vi "Untitled 2.vi"(7 "Before":dbl[][](array[numeric]), 11 "After":dbl[][](array[numeric])) -> (6 "Numeric":dbl)   [LabVIEW 2016]
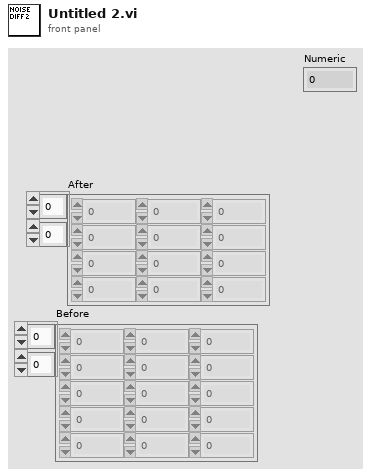
[diagram p1: front panel]
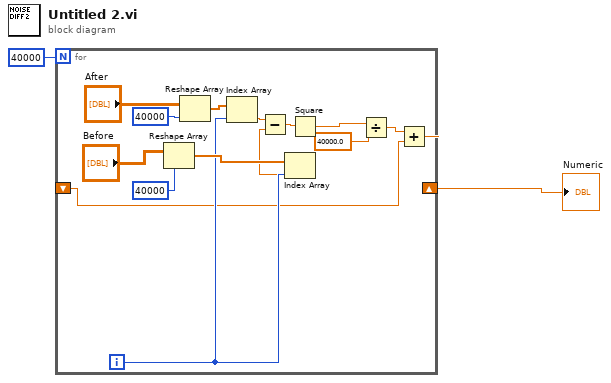
[diagram p0: block diagram]
diagram:
  n1 = for {
    N: 40000 -> [_]
    shift-right: [w7] -> w1
    shift-left: _ -> [w8]
    i -> [w11]
    n2 = Reshape Array("Before", 40000 ("dimension size")) -> (w12:dbl[])
    n3 = Reshape Array("After", 40000 ("dimension size")) -> (w13:dbl[])
    n4 = Index Array(array=w13, index=w11) -> (element=w10:dbl)
    n5 = Index Array(array=w12, index=w11) -> (element=w9:dbl)
    n6 = Subtract(x=w10, y=w9) -> (x-y=w6:dbl)
    n7 = Square(x=w6) -> (x^2=w4:dbl)
    n8 = Divide(x=w4, y=40000.0) -> (x/y=w3:dbl)
    n9 = Add(x=w3, y=w8) -> (x+y=w7:dbl)
  }
  "Numeric" <- w1
